vi "Public Application Data Text File Sink.vi"(7 "Log Level":T1) -> (3 "Text File Sink":refnum<class "Text File Sink.lvclass">)   [LabVIEW 2017, in "EventSinkConfigurations.lvlib"]
uses:
  EventSinkConfigurations.lvlib
  gpm_packages/@cs/event-logger/Source/Text File Sink/Text File Sink.lvclass
  gpm_packages/@cs/event-logger/Source/Composed Log/Log Sink/Log Level.ctl
  <vilib>/Utility/sysdir.llb/System Directory Type.ctl
  gpm_packages/@cs/event-logger/Source/Composed Log/Log Sink/Log Sink.lvclass
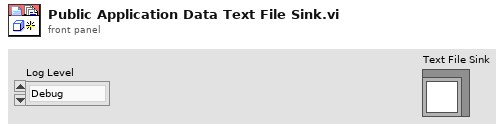
[diagram p1: front panel]
types:
  T1 = typedef "Composed Log.lvlib/Log Sink.lvclass/Log Level.ctl" = enum16{"Debug", "Info", "Warning", "Error", "Critical"}
  T2 = typedef "System Directory Type.ctl" = i32
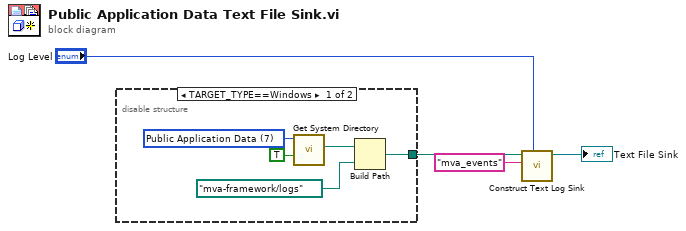
[diagram p0: block diagram]
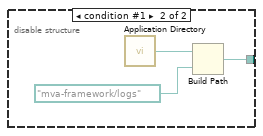
[diagram p2: hidden frame]
diagram:
  n1 = disable-structure shown="TARGET_TYPE==Windows" {
    disable-tunnel: [w6 w11] -> w3
    frame condition #0 (active) {
      w9 = T2 7 items=["User Home"=0, "User Desktop"=1, "User Documents"=2, "User Application Data"=3, "User Preferences"=4, "User Temporary"=5, "Public Documents"=6, "Public Application Data"=7, "Public Preferences"=8, "Public Cache"=13, "System Core Libraries"=9, "System Installed Libraries"=10, "Application Files"=11, "Boot Volume Root"=12] ("system directory type")
      n2 = call <vilib>:"Get System Directory.vi"("create directory if not found? (F)"=TRUE, "system directory type"=w9) -> ("system directory"=w7:path)  [unwired: 9 in]
      n3 = Build Path(base path=w7, name or relative path=path "mva-framework/logs") -> (appended path=w6:path)
    }
    frame condition #1 {
      n4 = call <vilib>:"Application Directory.vi"() -> ("Application Directory"=w10:path)
      n5 = Build Path(base path=w10, name or relative path=path "mva-framework/logs") -> (appended path=w11:path)
    }
  }
  n6 = call "Construct Text Log Sink.vi"("LogLevel"="Log Level", "File Name"="mva_events", "Log File Folder"=w3) -> ("Text File Sink out"=→"Text File Sink":refnum<class "Text File Sink.lvclass">)  [unwired: 8 in]
